vi "Save Class for Previous.vi"() -> ()   [LabVIEW 2020]
uses:
  source/Session/Session.lvclass
panel:
  out "error out":errorcluster
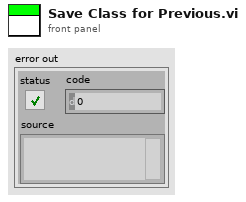
[diagram p1: front panel]
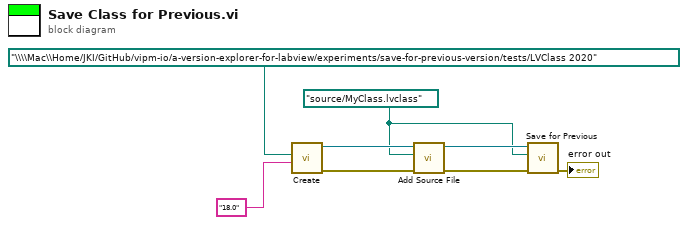
[diagram p0: block diagram]
diagram:
  w2 = path "source/MyClass.lvclass" ("Source File")
  n1 = call "Create.vi"("LabVIEW Version"="18.0", "Source Folder"=path "\\\\Mac\\Home/JKI/GitHub/vipm-io/a-version-explorer-for-labview/experiments/save-for-previous-version/tests/LVClass 2020" ("Path")) -> ("error out"=w5:errorcluster, "Session out"=w6:refnum<class "Session.lvclass">)  [unwired: 8 in]
  n2 = call "Add Source File.vi"("error in (no error)"=w5, "Source File"=w2, "Session in"=w6) -> ("error out"=w4:errorcluster, "Session out"=w3:refnum<class "Session.lvclass">)  [unwired: 7 in]
  n3 = call "Save for Previous.vi"("error in (no error)"=w4, "File Path"=w2, "Session in"=w3) -> ("error out"=→"error out":errorcluster)  [unwired: 7 in, 1 out]
